vi "DynamixelReadPosition.vi"() -> ()   [LabVIEW 2013]
uses:
  <instrlib>/Dynamixel Motor/Dynamixel Motor.lvlib
panel:
  in  "stop":bool
  out "Array":dbl[](array[numeric])
  out "Motors IDs Found":u8[](array[numeric])
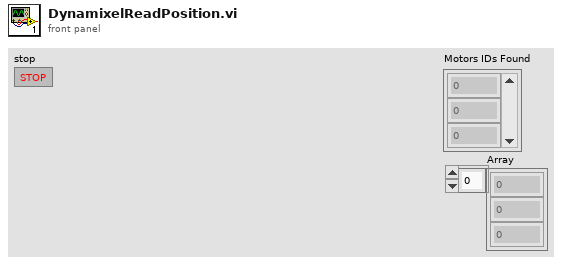
[diagram p1: front panel]
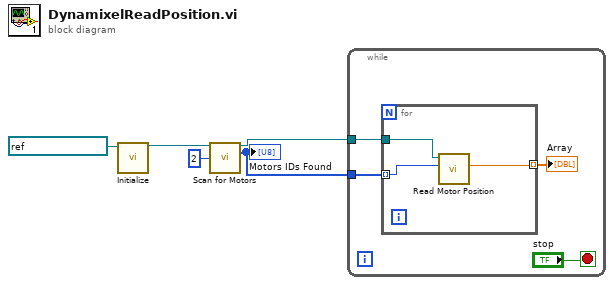
[diagram p0: block diagram]
diagram:
  n1 = call <instrlib>:"Initialize.vi"("VISA resource name"=refnum<visa-resource-name> "ASRL3::INSTR") -> ("VISA resource name out"=w4:refnum<visa-resource-name>)  [unwired: 9 in, 1 out]
  n2 = call <instrlib>:"Scan for Motors.vi"("VISA resource name"=w4, "Ending ID (253)"=u8 2) -> ("VISA resource name out"=w1:refnum<visa-resource-name>, "Motors IDs Found"=w2:u8[])  [unwired: 11 in, 1 out]
  "Motors IDs Found" <- w2
  n3 = while {
    tunnel: w2 -> [w9]
    tunnel: w1 -> [w8]
    stop <- "stop" stop-if-true
    n4 = for {
      tunnel: w9 -> [w12] mode=indexing
      tunnel: w8 -> [w11]
      tunnel: [w10] -> w7 mode=indexing
      n5 = call <instrlib>:"Read Motor Position.vi"("Motor ID (0)"=w12, "VISA resource name"=w11) -> ("Position (deg)"=w10:dbl)  [unwired: 7 in, 2 out]
    }
    "Array" <- w7
  }
